vi "Temp Ramp Rate--SubVI.vi"(4 "Instance(1)":i32=1, 6 "Temp Ramp Data":T1, 8 "error in (no error)":errorcluster, 10 "Get/Set":enum16{"Get", "Set"}(ring), 11 "Watlow F4T in":refnum<class "Watlow F4T.lvclass">) -> (0 "error out":errorcluster, 2 "Temp Ramp Rate":dbl, 3 "Watlow F4T out":refnum<class "Watlow F4T.lvclass">)   [LabVIEW 2024, in "Watlow F4T.lvclass"]
uses:
  Watlow F4T.lvclass
  Process Controller/Controls/Temp Ramp Rate Data--Cluster.ctl
  Process Controller/Controls/Temperature Units--Enum.ctl
  Process Controller/Controls/Rate Units--Enum.ctl
  Private/Controls/Standard Bus Commands--Enum.ctl
  Process Controller/_Thermal Process Controller.lvclass
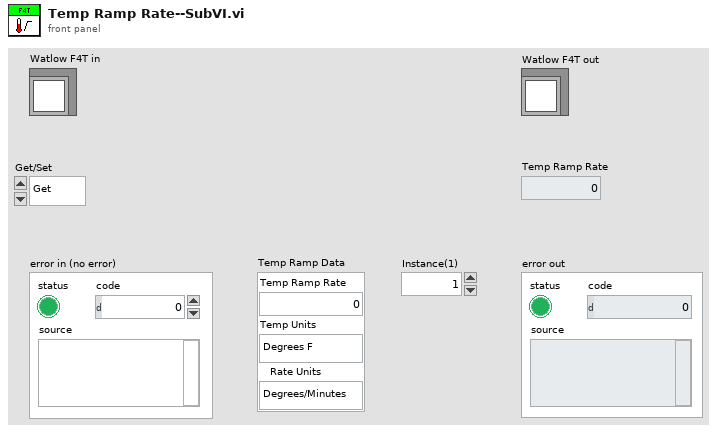
[diagram p1: front panel]
types:
  T1 = typedef "_Thermal Process Controller.lvclass/Temp Ramp Rate Data--Cluster.ctl" = cluster{"Temp Ramp Rate":dbl, "Temp Units":T2, "Rate Units":T3}
  T2 = typedef "_Thermal Process Controller.lvclass/Temperature Units--Enum.ctl" = enum16{"Degrees F", "Degrees C", "Degrees K"}
  T3 = typedef "_Thermal Process Controller.lvclass/Rate Units--Enum.ctl" = enum16{"Degrees/Minutes", "Degrees/Hours"}
  T4 = typedef "Watlow F4T.lvclass/Standard Bus Commands--Enum.ctl" = enum16{"Remote Setpoint", "Remote Mode", "Temp Feedback", "Target Setpoint", "Current Setpoint", "Setpoint Lower Limit", "Setpoint Upper Limit", "Ramp Rate Y", "Ramp Rate X", "Ramp Rate Action", "Temp Control State", "Temp Control Mode", "Power", "Heat Power", "Cool Power"}
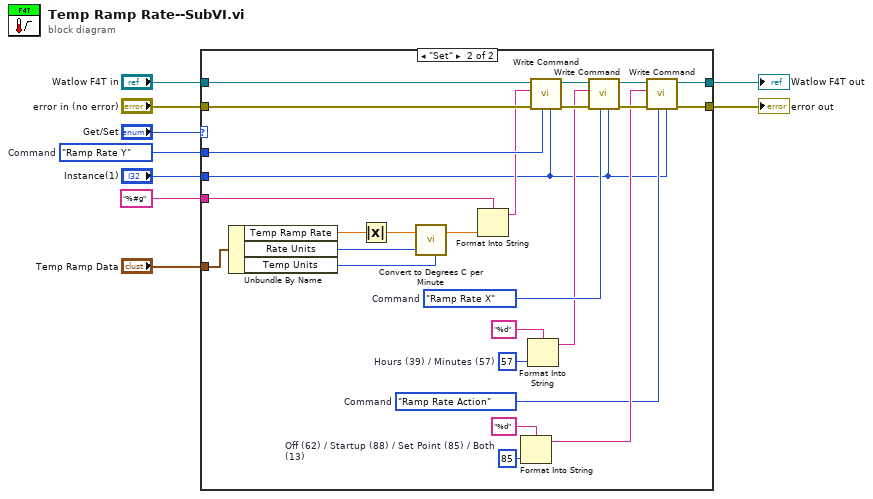
[diagram p0: block diagram]
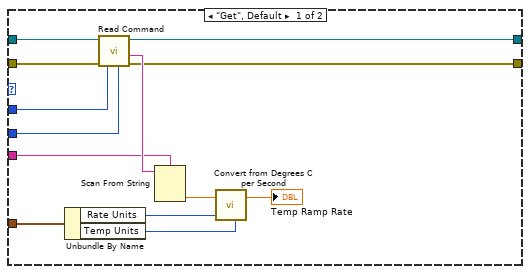
[diagram p2: hidden frame]
diagram:
  w5 = Standard_Bus_Commands--Enum."Ramp Rate Y"  # Command
  n1 = case shown="\"Set\"" "Get/Set" {
    tunnel: [w15 w28] -> w9
    tunnel: "%#g" ("format string") -> [w19 w40]
    tunnel: "Instance(1)" -> [w21 w23]
    tunnel: w5 -> [w22 w39]
    tunnel: "Temp Ramp Data" -> [w17 w37]
    tunnel: [w11 w26] -> w3
    tunnel: "Watlow F4T in" -> [w13 w34]
    tunnel: "error in (no error)" -> [w12 w33]
    frame "Get", Default {
      n2 = Unbundle By Name(w17) -> ("Rate Units"=w10:T3, "Temp Units"=w16:T2)
      n3 = call "Read Command.vi"("Instance"=w21, "Commands"=w22, "error in (no error)"=w12, "Watlow F4T In"=w13) -> ("error out"=w15:errorcluster, "Value Out"=w20:string, "Watlow F4T out"=w11:refnum<class "Watlow F4T.lvclass">)  [unwired: 5 in]
      n4 = Scan From String(format string=w19, input string=w20) -> (output 1=w18:dbl)  [unwired: 3 in, 3 out]
      n5 = call "Convert from Degrees C per Second.vi"("Rate In"=w18, "Rate Units"=w10, "Temp Units"=w16) -> ("Rate Out"=→"Temp Ramp Rate":dbl)  [unwired: 4 in]
    }
    frame "Set" {
      w29 = 85  # Off (62) / Startup (88) / Set Point (85) / Both (13)
      w24 = Standard_Bus_Commands--Enum."Ramp Rate Action"  # Command
      w35 = Standard_Bus_Commands--Enum."Ramp Rate X"  # Command
      w38 = 57  # Hours (39) / Minutes (57)
      n6 = Unbundle By Name(w37) -> ("Temp Ramp Rate"=w43:dbl, "Rate Units"=w42:T3, "Temp Units"=w41:T2)
      n7 = Absolute Value(x=w43) -> (abs(x)=w46:dbl)
      n8 = call "Convert to Degrees C per Minute.vi"("Rate In"=w46, "Rate Units"=w42, "Temp Units"=w41) -> ("Rate Out"=w48:dbl)  [unwired: 4 in]
      n9 = Format Into String(format string=w40, w48) -> (resulting string=w32:string)  [unwired: 2 in, 1 out]
      n10 = Format Into String(format string="%d", w29) -> (resulting string=w25:string)  [unwired: 2 in, 1 out]
      n11 = Format Into String(format string="%d", w38) -> (resulting string=w31:string)  [unwired: 2 in, 1 out]
      n12 = call "Write Command.vi"("Instance"=w23, "Commands"=w39, "error in (no error)"=w33, "Set Value"=w32, "Watlow F4T In"=w34) -> ("error out"=w44:errorcluster, "Watlow F4T out"=w45:refnum<class "Watlow F4T.lvclass">)  [unwired: 5 in]
      n13 = call "Write Command.vi"("Instance"=w23, "Commands"=w35, "error in (no error)"=w44, "Set Value"=w31, "Watlow F4T In"=w45) -> ("error out"=w47:errorcluster, "Watlow F4T out"=w27:refnum<class "Watlow F4T.lvclass">)  [unwired: 5 in]
      n14 = call "Write Command.vi"("Instance"=w23, "Commands"=w24, "error in (no error)"=w47, "Set Value"=w25, "Watlow F4T In"=w27) -> ("error out"=w28:errorcluster, "Watlow F4T out"=w26:refnum<class "Watlow F4T.lvclass">)  [unwired: 5 in]
    }
  }
  "error out" <- w9
  "Watlow F4T out" <- w3
